vi "FindOrAddGUIDSubchannel.vi"(8 "GUID":string, 11 "MessengerMCPU in":refnum<class "MessengerMCPU.lvclass">) -> (0 "GUIDsubchannel":i32, 3 "MessengerMCPU out":refnum<class "MessengerMCPU.lvclass">)   [LabVIEW 2019, in "MessengerM.lvlib" / "MessengerMCPU.lvclass"]
uses:
  MessengerMCPU.lvclass
  SubChannelCPU/SubChannelCPU.lvclass
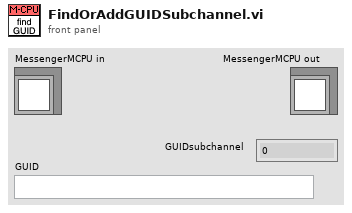
[diagram p1: front panel]
types:
  T1 = cluster{"GUID":string, "sub":refnum<class "SubChannelCPU.lvclass">}[]
  T2 = cluster{"GUID":string, "SubChannel out":refnum<class "SubChannelCPU.lvclass">}
  T3 = cluster{"GUID":string, "SubChannel out":refnum<class "SubChannelCPU.lvclass">}[]
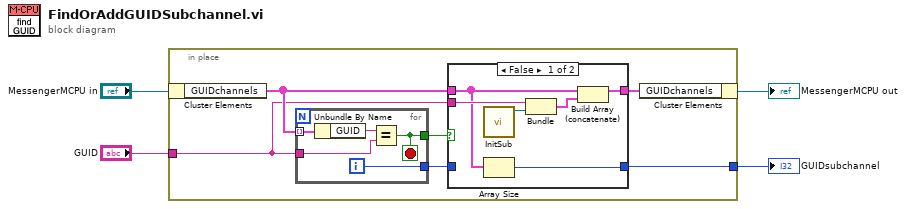
[diagram p0: block diagram]
diagram:
  n1 = in-place {
    in-place-border: "GUID" -> [w5]
    in-place-border: [w9] -> w1
    n2 = in-place-cluster #1("MessengerMCPU in") -> ("GUIDchannels"=w6:T1)
    n3 = for {
      tunnel: w6 -> [w15] mode=indexing
      tunnel: w5 -> [w13]
      tunnel: [w12] -> w10
      tunnel: [w11] -> w8
      i -> [w11]
      stop <- w12 stop-if-true
      n4 = Unbundle By Name(w15) -> ("GUID"=w14:string)
      n5 = Equal?(x=w14, y=w13) -> (x = y?=w12:bool)
    }
    n6 = case shown="False" w10 {
      tunnel: [w17 w23] -> w9
      tunnel: w8 -> [_ w23]
      tunnel: [w21 w22] -> w7
      tunnel: w6 -> [w18 w22]
      tunnel: w5 -> [w20 _]
      frame False {
        n7 = call "InitSub.vi"() -> ("SubChannel out"=w16:refnum<class "SubChannelCPU.lvclass">)  [unwired: 11 in]
        n8 = Array Size(array=w18) -> (size(s)=w17:i32)
        n9 = Bundle("GUID"=w20, "SubChannel out"=w16) -> (w19:T2)  [unwired: 1 in]
        n10 = Build Array (concatenate)(w18, w19) -> (w21:T3)
      }
      frame True {
      }
    }
    n11 = in-place-cluster #1("GUIDchannels"=w7) -> (→"MessengerMCPU out":refnum<class "MessengerMCPU.lvclass">)
  }
  "GUIDsubchannel" <- w1
